vi "IECMemory.ProcCases.vi"(0 "i ref in":refnum<vi>, 1 "selector":string, 2 "Data":T2, 3 "call cluster":T6={"Object"="", "Selector"="", "CallType"=enum."synchronous", "Async Object"="", "Async Selector"="", "Data Descriptor"="", "Data"=[], "Error #"=0, "Expire"=0}, 5 "error in (no error)":errorcluster) -> (14 "i ref out":refnum<vi>, 17 "answer cluster":T6={"Object"="", "Selector"="", "CallType"=enum."synchronous", "Async Object"="", "Async Selector"="", "Data Descriptor"="", "Data"=[], "Error #"=0, "Expire"=0}, 19 "error out":errorcluster)   [LabVIEW 2014, in "IECMemory.lvlib"]
doc: "This method is called by a process from within the default case in the event loop. The methods of a class that are linked to events will be called from THIS method. Add your code here."
uses:
  IECMemory.lvlib
  CS_Core/BaseProcess/BaseProcess.lvlib
  CS_Core/CSSystem/CoreLib/CoreLib.lvlib
  CS_Core/CSSystem/CoreLib/CoreLib.string 2 byte array.vi
  CS_Core/CSSystem/CoreLib/CoreLib.byte array 2 string.vi
  CS_Core/CSSystem/CoreLib/CoreLib.byte array 2 int.vi
  CS_Core/CSSystem/CoreDefs/CoreDefs.call_type.ctl
  instr.lib/GPIB_Memory/Memory_Status.ctl
  CS_Lebit/LEBITDefs/LEBITDefs.MemDevInfo.ctl
  CS_Lebit/LEBITDefs/LEBITDefs.lvlib
  CS_Core/BaseProcess/BaseProcess.descriptor string definition.ctl
  CS_Core/CSSystem/CoreDefs/CoreDefs.rawDataType.ctl
  CS_Lebit/LEBITDefs/LEBITDefs.Memory.ctl
  CS_Lebit/LEBITDefs/LEBITDefs.Timetable.ctl
panel:
  in  "MemoryStatusBits":T1=[TRUE]
  in  "ms timeout (100)":i32=100
  in  "MemDevInfo":T3
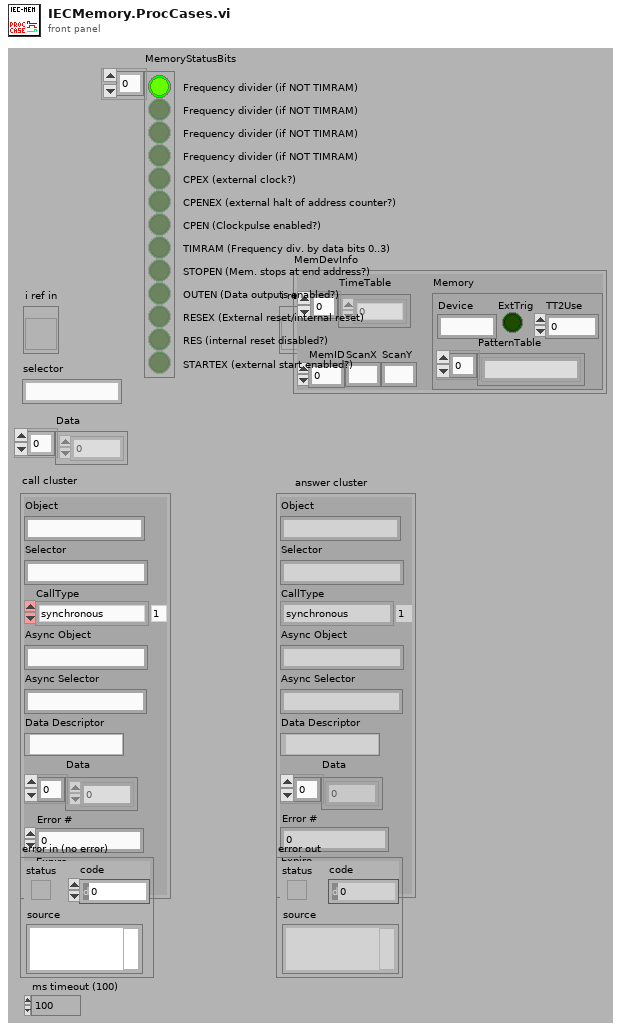
[diagram p1: front panel]
types:
  T1 = typedef "IECMemoryDriver.lvlib/Memory_Status.ctl" = bool[]
  T2 = typedef "CoreDefs.rawDataType.ctl" = i8[]
  T3 = typedef "LEBITDefs.lvlib/LEBITDefs.MemDevInfo.ctl" = cluster{"TimeTable":T4, "Memory":T5, "MemID":i32, "ScanX":string, "ScanY":string}
  T4 = typedef "LEBITDefs.lvlib/LEBITDefs.Timetable.ctl" = dbl[]
  T5 = typedef "LEBITDefs.lvlib/LEBITDefs.Memory.ctl" = cluster{"Device":string, "ExtTrig":bool, "TT2Use":i32, "PatternTable":string[]}
  T6 = typedef "CoreDefs.call_type.ctl" = cluster{"Object":string, "Selector":string, "CallType":enum16{"simple", "synchronous", "asynchronous"}, "Async Object":string, "Async Selector":string, "Data Descriptor":T7, "Data":T2, "Error #":i32, "Expire":u32}
  T7 = typedef "BaseProcess.lvlib/BaseProcess.descriptor string definition.ctl" = string
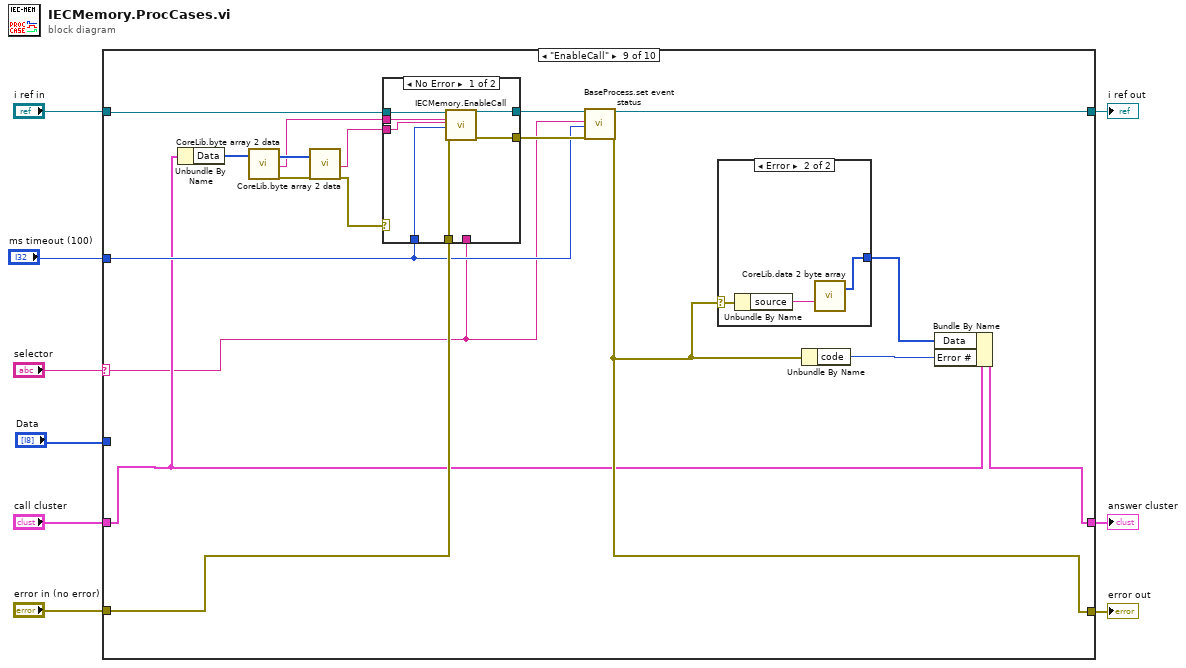
[diagram p0: block diagram]
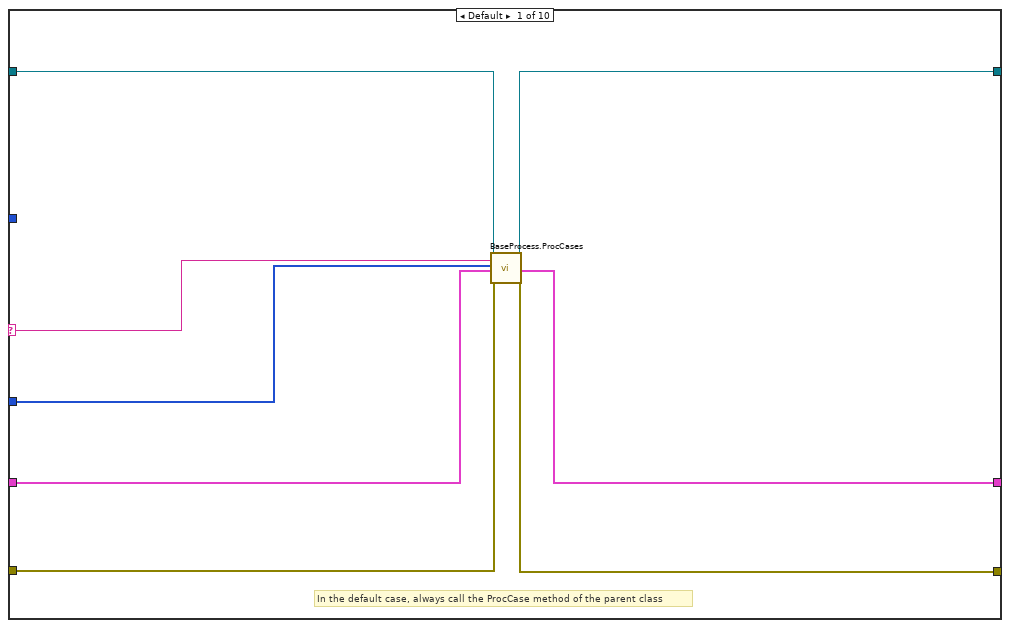
[diagram p2: hidden frame]
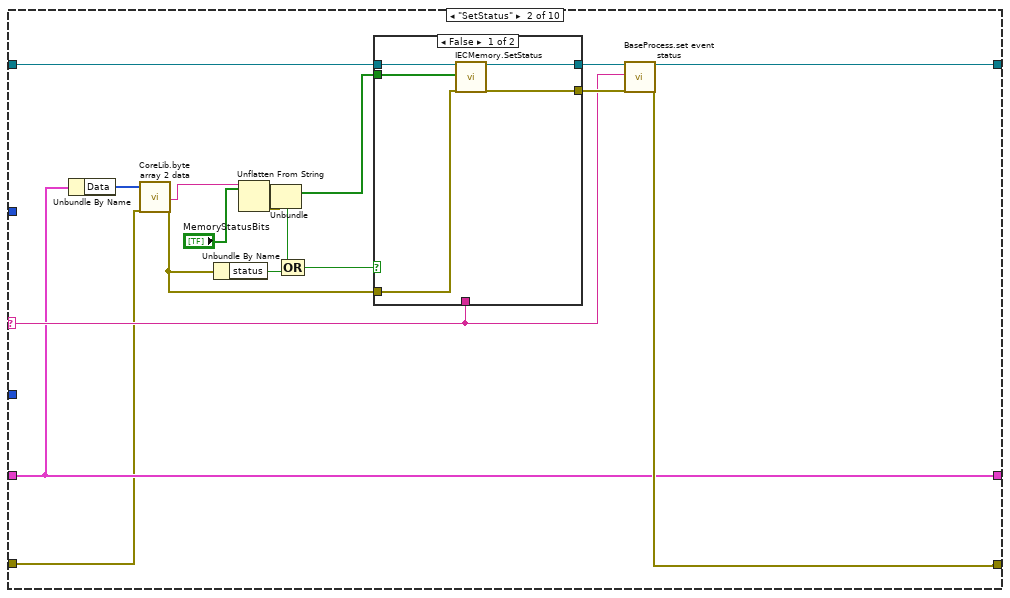
[diagram p3: hidden frame]
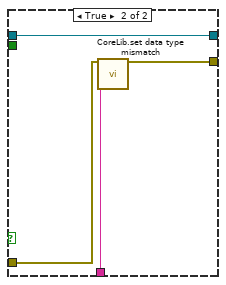
[diagram p4: hidden frame]
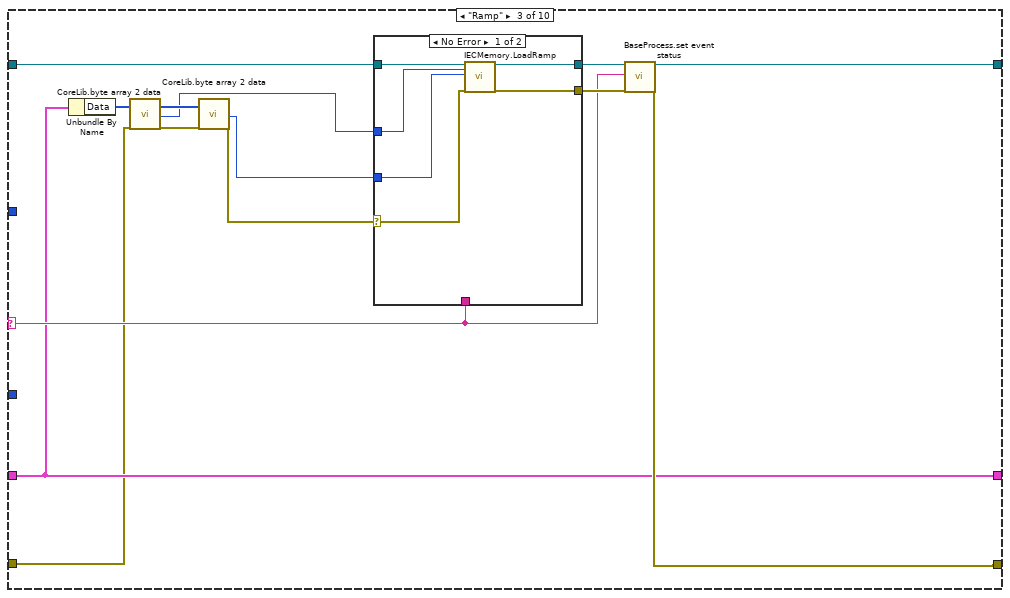
[diagram p5: hidden frame]
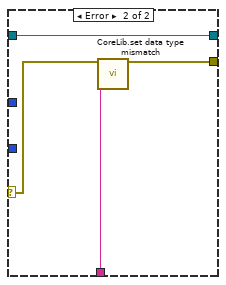
[diagram p6: hidden frame]
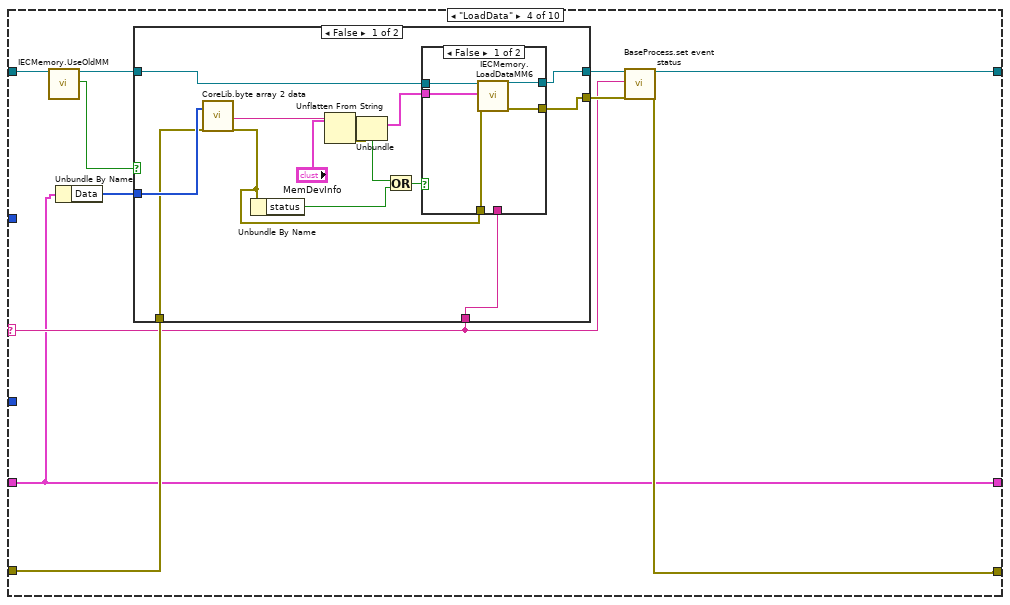
[diagram p7: hidden frame]
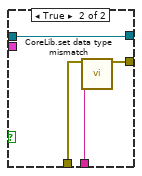
[diagram p8: hidden frame]
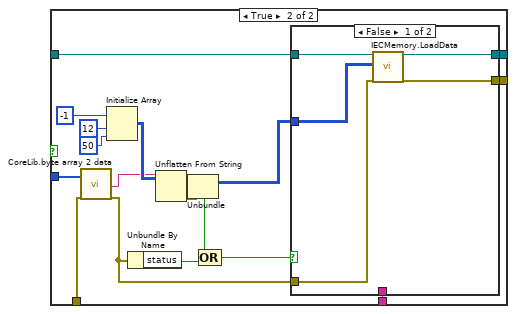
[diagram p9: hidden frame]
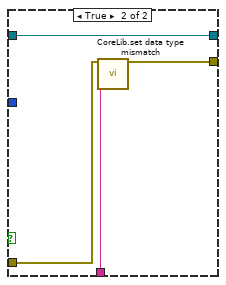
[diagram p10: hidden frame]
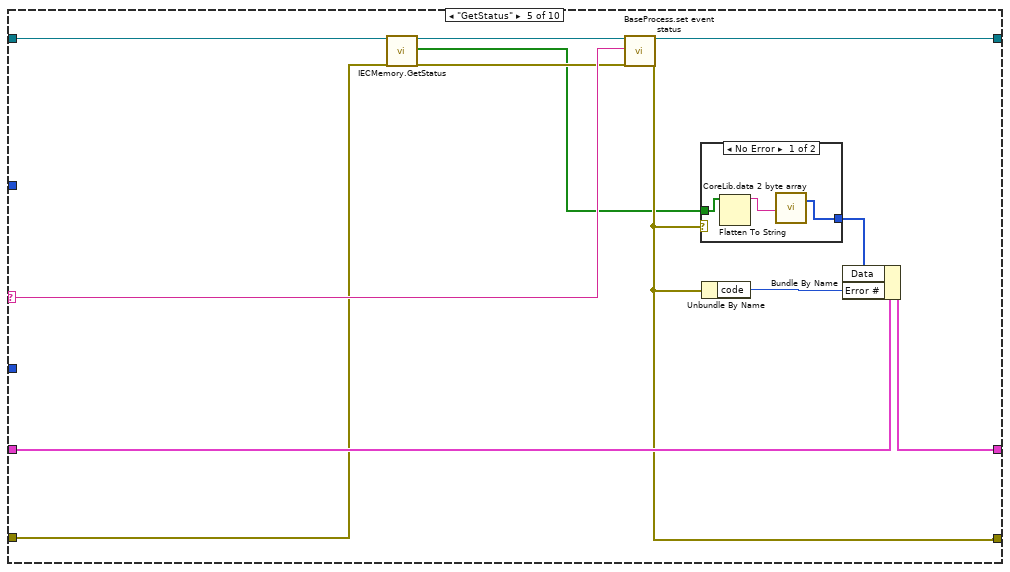
[diagram p11: hidden frame]
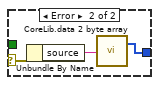
[diagram p12: hidden frame]
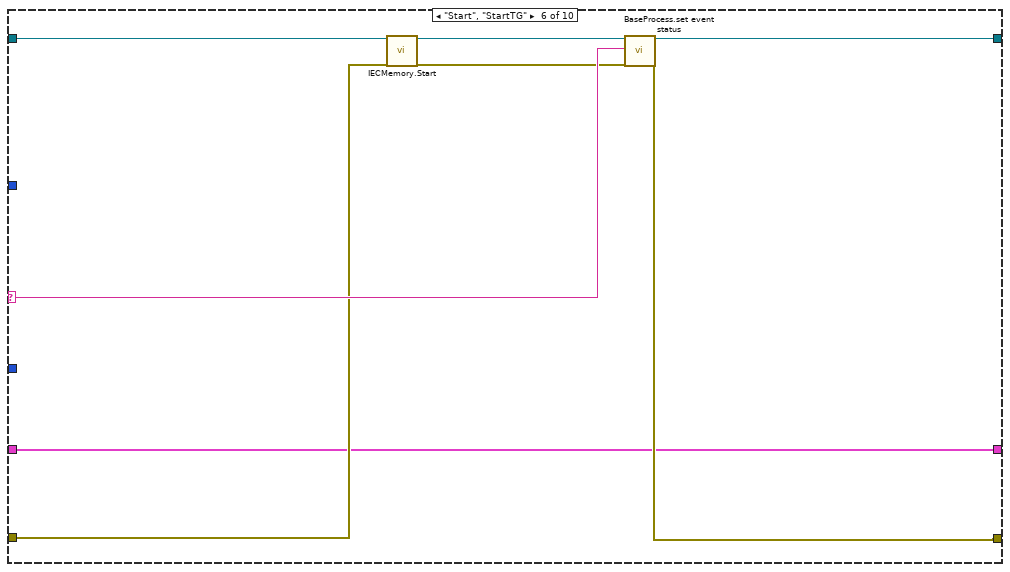
[diagram p13: hidden frame]
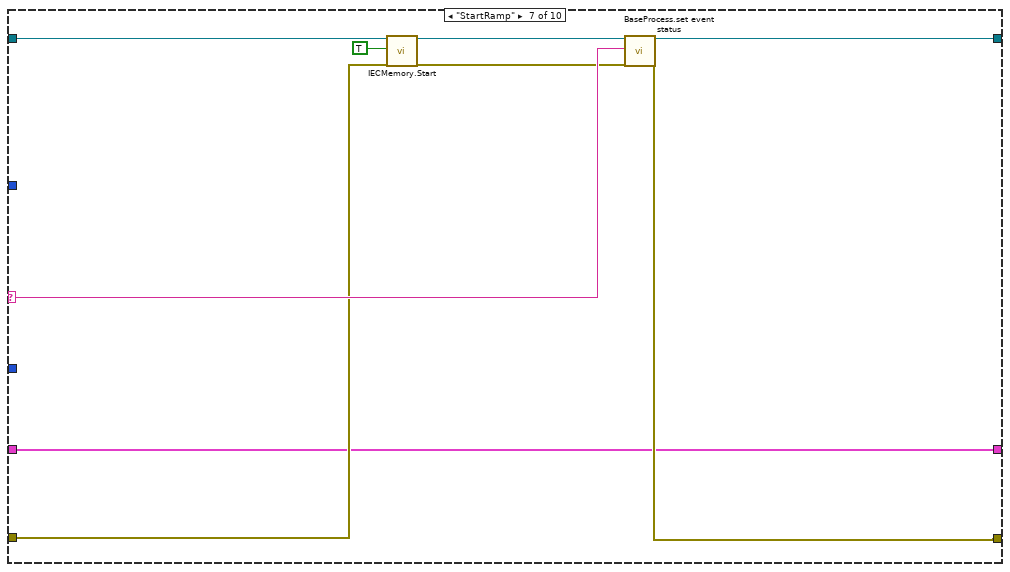
[diagram p14: hidden frame]
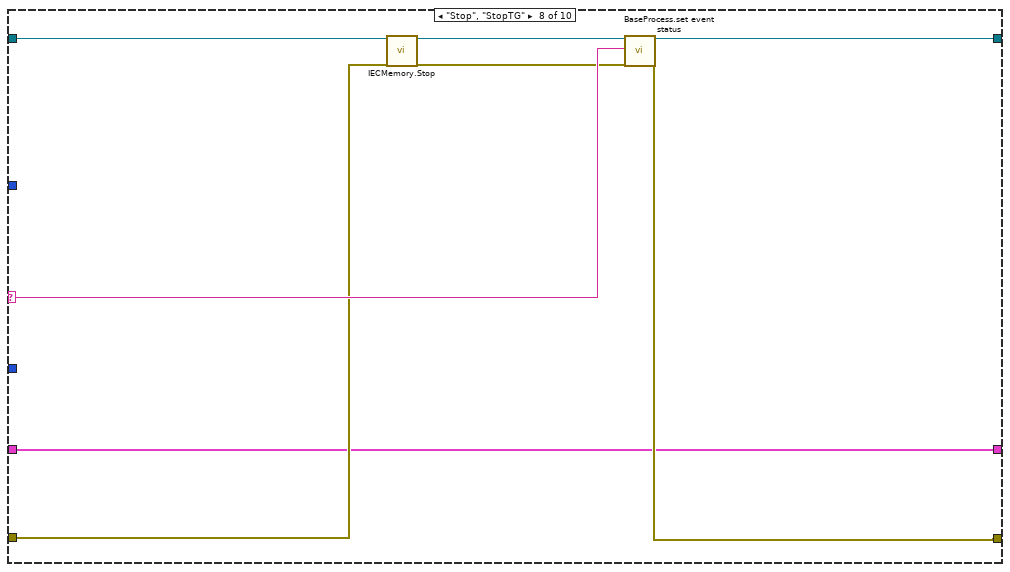
[diagram p15: hidden frame]
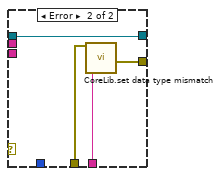
[diagram p16: hidden frame]
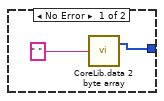
[diagram p17: hidden frame]
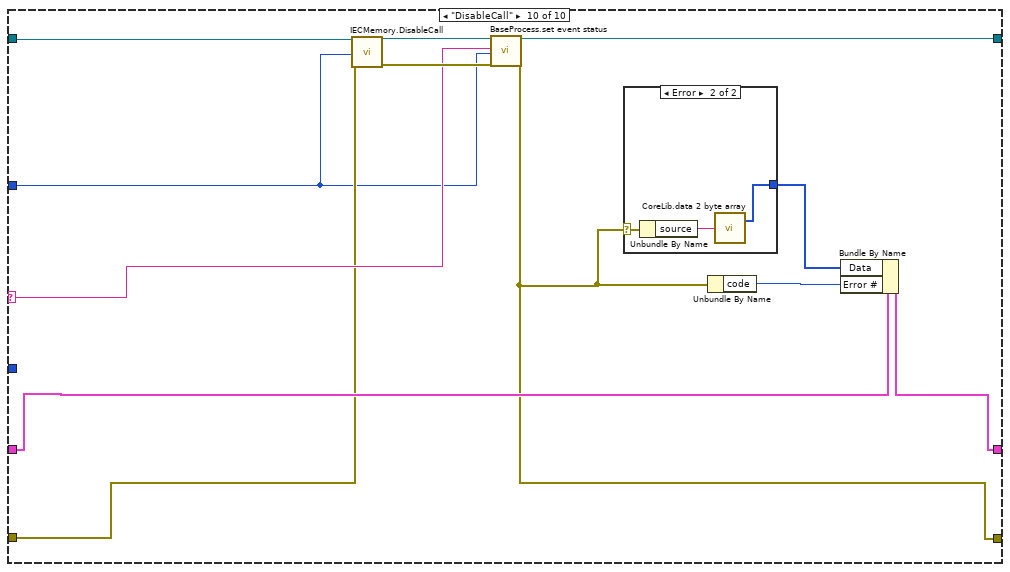
[diagram p18: hidden frame]
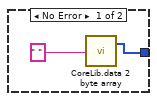
[diagram p19: hidden frame]
diagram:
  n1 = case shown="\"EnableCall\"" "selector" {
    selector: "selector" -> [w11 w29 w54 w75 w135 w152 w161 w169 w177 w210]
    tunnel: "Data" -> [w12 _ _ _ _ _ _ _ _ _]
    tunnel: "i ref in" -> [w10 w32 w57 w70 w133 w150 w159 w167 w184 w212]
    tunnel: [w17 w27 w53 w74 w134 w151 w160 w168 w182 w208] -> w5
    tunnel: "call cluster" -> [w13 w25 w51 w72 w138 w146 w155 w163 w178 w211]
    tunnel: [w14 w25 w51 w72 w137 w146 w155 w163 w181 w207] -> w8
    tunnel: "error in (no error)" -> [w16 w20 w44 w78 w132 w149 w158 w166 w183 w209]
    tunnel: [w15 w26 w52 w73 w136 w153 w162 w170 w180 w206] -> w3
    tunnel: "ms timeout (100)" -> [_ _ _ _ _ _ _ _ w179 w205]
    frame Default {
      # "In the default case, always call the ProcCase method of the parent class"
      n2 = call "BaseProcess.ProcCases.vi"("i ref in"=w10, "selector"=w11, "Data"=w12, "call cluster"=w13, "error in (no error)"=w16) -> ("i ref out"=w17:refnum<vi>, "answer cluster"=w14:T6, "error out"=w15:errorcluster)  [unwired: 12 in]
    }
    frame "SetStatus" {
      n3 = Unbundle By Name(w25) -> ("Data"=w24:T2)
      n4 = call-poly "CoreLib.byte array 2 data.vi"("byteArray"=w24, "error in (no error)"=w20) -> ("string"=w23:string, "error out"=w21:errorcluster)  [unwired: 15 in, 1 out]
      n5 = Unbundle By Name(w21) -> ("status"=w22:bool)
      n6 = Unflatten From String(type="MemoryStatusBits", binary string=w23) -> (value=w28:T1, error out=w18:errorcluster)  [unwired: 3 in, 1 out]
      n7 = Unbundle(w18) -> ("status"=w34:bool)  [unwired: 2 out]
      n8 = Compound Arithmetic op=OR(w34, w22) -> (w33:bool)
      n9 = case shown="False" w33 {
        tunnel: [w37 w43] -> w31
        tunnel: w32 -> [w38 w43]
        tunnel: [w36 w42] -> w30
        tunnel: w29 -> [_ w41]
        tunnel: w28 -> [w39 _]
        tunnel: w21 -> [w35 w40]
        frame False {
          n10 = call "IECMemory.SetStatus.vi"("i ref in"=w38, "MemoryStatusBits"=w39, "error in (no error)"=w35) -> ("i ref out"=w37:refnum<vi>, "error out"=w36:errorcluster)  [unwired: 14 in, 1 out]
        }
        frame True {
          n11 = call "CoreLib.set data type mismatch.vi"("error in (no error)"=w40, "error source"=w41) -> ("error out"=w42:errorcluster)  [unwired: 17 in]
        }
      }
      n12 = call "BaseProcess.set event status.vi"("i ref in"=w31, "EventStatus"=w29, "error in (no error)"=w30) -> ("i ref out"=w27:refnum<vi>, "error out"=w26:errorcluster)  [unwired: 14 in, 1 out]
    }
    frame "Ramp" {
      n13 = Unbundle By Name(w51) -> ("Data"=w50:T2)
      n14 = call-poly "CoreLib.byte array 2 data.vi"("byteArray"=w50, "error in (no error)"=w44) -> ("byteArray out"=w49:T2, "i32"=w45:i32, "error out"=w48:errorcluster)  [unwired: 15 in]
      n15 = call-poly "CoreLib.byte array 2 data.vi"("byteArray"=w49, "error in (no error)"=w48) -> ("i32"=w46:i32, "error out"=w47:errorcluster)  [unwired: 15 in, 1 out]
      n16 = case shown="No Error" w47 {
        selector: w47 -> [w58 w64]
        tunnel: [w62 w67] -> w56
        tunnel: w57 -> [w63 w67]
        tunnel: [w61 w66] -> w55
        tunnel: w54 -> [_ w65]
        tunnel: w45 -> [w59 _]
        tunnel: w46 -> [w60 _]
        frame No Error {
          n17 = call "IECMemory.LoadRamp.vi"("i ref in"=w63, "FirstStep"=w59, "SecondStep"=w60, "error in (no error)"=w58) -> ("i ref out"=w62:refnum<vi>, "error out"=w61:errorcluster)  [unwired: 13 in, 1 out]
        }
        frame Error {
          n18 = call "CoreLib.set data type mismatch.vi"("error in (no error)"=w64, "error source"=w65) -> ("error out"=w66:errorcluster)  [unwired: 17 in]
        }
      }
      n19 = call "BaseProcess.set event status.vi"("i ref in"=w56, "EventStatus"=w54, "error in (no error)"=w55) -> ("i ref out"=w53:refnum<vi>, "error out"=w52:errorcluster)  [unwired: 14 in, 1 out]
    }
    frame "LoadData" {
      n20 = call "IECMemory.UseOldMM.vi"("i ref in"=w70) -> ("i ref out"=w69:refnum<vi>, "Use Old MM?"=w68:bool)  [unwired: 15 in, 2 out]
      n21 = Unbundle By Name(w72) -> ("Data"=w71:T2)
      n22 = case shown="False" w68 {
        tunnel: w69 -> [w88 w116]
        tunnel: w78 -> [w81 w107]
        tunnel: [w90 w115] -> w77
        tunnel: [w89 w114] -> w76
        tunnel: w75 -> [w87 w113]
        tunnel: w71 -> [w86 w105]
        frame False {
          n23 = call-poly "CoreLib.byte array 2 data.vi"("byteArray"=w86, "error in (no error)"=w81) -> ("string"=w85:string, "error out"=w80:errorcluster)  [unwired: 15 in, 1 out]
          n24 = Unbundle By Name(w80) -> ("status"=w82:bool)
          n25 = Unflatten From String(type="MemDevInfo", binary string=w85) -> (value=w92:T3, error out=w79:errorcluster)  [unwired: 3 in, 1 out]
          n26 = Unbundle(w79) -> ("status"=w83:bool)  [unwired: 2 out]
          n27 = Or(x=w83, y=w82) -> (x .or. y?=w84:bool)
          n28 = case shown="False" w84 {
            tunnel: w88 -> [w97 w99]
            tunnel: w80 -> [w96 w100]
            tunnel: [w95 w99] -> w90
            tunnel: [w94 w101] -> w89
            tunnel: w92 -> [w93 _]
            tunnel: w87 -> [_ w98]
            frame False {
              n29 = call "IECMemory.LoadDataMM6.vi"("i ref in"=w97, "MemDevInfo"=w93, "error in (no error)"=w96) -> ("i ref out"=w95:refnum<vi>, "error out"=w94:errorcluster)  [unwired: 14 in, 1 out]
            }
            frame True {
              n30 = call "CoreLib.set data type mismatch.vi"("error in (no error)"=w100, "error source"=w98) -> ("error out"=w101:errorcluster)  [unwired: 17 in]
            }
          }
        }
        frame True {
          n31 = call-poly "CoreLib.byte array 2 data.vi"("byteArray"=w105, "error in (no error)"=w107) -> ("string"=w106:string, "error out"=w104:errorcluster)  [unwired: 15 in, 1 out]
          n32 = Initialize Array(-1 ("element"), 12 ("dimension size"), 50 ("dimension size")) -> (w108:i32[][])
          n33 = Unbundle By Name(w104) -> ("status"=w103:bool)
          n34 = Unflatten From String(type=w108, binary string=w106) -> (value=w112:i32[][], error out=w102:errorcluster)  [unwired: 3 in, 1 out]
          n35 = Unbundle(w102) -> ("status"=w118:bool)  [unwired: 2 out]
          n36 = Compound Arithmetic op=OR(w118, w103) -> (w117:bool)
          n37 = case shown="False" w117 {
            tunnel: [w122 w127] -> w115
            tunnel: w116 -> [w123 w127]
            tunnel: [w121 w126] -> w114
            tunnel: w113 -> [_ w125]
            tunnel: w112 -> [w120 _]
            tunnel: w104 -> [w119 w124]
            frame False {
              n38 = call "IECMemory.LoadData.vi"("i ref in"=w123, "MemoryTimingArray"=w120, "error in (no error)"=w119) -> ("i ref out"=w122:refnum<vi>, "error out"=w121:errorcluster)  [unwired: 14 in, 1 out]
            }
            frame True {
              n39 = call "CoreLib.set data type mismatch.vi"("error in (no error)"=w124, "error source"=w125) -> ("error out"=w126:errorcluster)  [unwired: 17 in]
            }
          }
        }
      }
      n40 = call "BaseProcess.set event status.vi"("i ref in"=w77, "EventStatus"=w75, "error in (no error)"=w76) -> ("i ref out"=w74:refnum<vi>, "error out"=w73:errorcluster)  [unwired: 14 in, 1 out]
    }
    frame "GetStatus" {
      n41 = call "IECMemory.GetStatus.vi"("i ref in"=w133, "error in (no error)"=w132) -> ("i ref out"=w131:refnum<vi>, "MemoryStatus"=w128:T1, "error out"=w130:errorcluster)  [unwired: 14 in, 1 out]
      n42 = call "BaseProcess.set event status.vi"("i ref in"=w131, "EventStatus"=w135, "error in (no error)"=w130) -> ("i ref out"=w134:refnum<vi>, "error out"=w136:errorcluster)  [unwired: 14 in, 1 out]
      n43 = case shown="No Error" w136 {
        selector: w136 -> [_ w145]
        tunnel: [w140 w143] -> w129
        tunnel: w128 -> [w142 _]
        frame No Error {
          n44 = Flatten To String(anything=w142) -> (data string=w141:string)  [unwired: 3 in, 2 out]
          n45 = call-poly "CoreLib.data 2 byte array.vi"("string"=w141) -> ("byteArray out"=w140:T2)  [unwired: 18 in]
        }
        frame Error {
          n46 = Unbundle By Name(w145) -> ("source"=w144:string)
          n47 = call-poly "CoreLib.data 2 byte array.vi"("string"=w144) -> ("byteArray out"=w143:T2)  [unwired: 18 in]
        }
      }
      n48 = Unbundle By Name(w136) -> ("code"=w139:i32)
      n49 = Bundle By Name(cluster=w138, "Data"=w129, "Error #"=w139) -> (w137:T6)
    }
    frame "Start", "StartTG" {
      n50 = call "IECMemory.Start.vi"("i ref in"=w150, "error in (no error)"=w149) -> ("i ref out"=w148:refnum<vi>, "error out"=w147:errorcluster)  [unwired: 15 in, 1 out]
      n51 = call "BaseProcess.set event status.vi"("i ref in"=w148, "EventStatus"=w152, "error in (no error)"=w147) -> ("i ref out"=w151:refnum<vi>, "error out"=w153:errorcluster)  [unwired: 14 in, 1 out]
    }
    frame "StartRamp" {
      n52 = call "IECMemory.Start.vi"("i ref in"=w159, "Ramp (F)"=TRUE, "error in (no error)"=w158) -> ("i ref out"=w157:refnum<vi>, "error out"=w156:errorcluster)  [unwired: 14 in, 1 out]
      n53 = call "BaseProcess.set event status.vi"("i ref in"=w157, "EventStatus"=w161, "error in (no error)"=w156) -> ("i ref out"=w160:refnum<vi>, "error out"=w162:errorcluster)  [unwired: 14 in, 1 out]
    }
    frame "Stop", "StopTG" {
      n54 = call "IECMemory.Stop.vi"("i ref in"=w167, "error in (no error)"=w166) -> ("i ref out"=w165:refnum<vi>, "error out"=w164:errorcluster)  [unwired: 15 in, 1 out]
      n55 = call "BaseProcess.set event status.vi"("i ref in"=w165, "EventStatus"=w169, "error in (no error)"=w164) -> ("i ref out"=w168:refnum<vi>, "error out"=w170:errorcluster)  [unwired: 14 in, 1 out]
    }
    frame "EnableCall" {
      n56 = Unbundle By Name(w178) -> ("Data"=w176:T2)
      n57 = call-poly "CoreLib.byte array 2 data.vi"("byteArray"=w176) -> ("byteArray out"=w174:T2, "string"=w172:string, "error out"=w175:errorcluster)  [unwired: 16 in]
      n58 = call-poly "CoreLib.byte array 2 data.vi"("byteArray"=w174, "error in (no error)"=w175) -> ("string"=w171:string, "error out"=w173:errorcluster)  [unwired: 15 in, 1 out]
      n59 = case shown="No Error" w173 {
        tunnel: [w195 w196] -> w186
        tunnel: [w194 w199] -> w185
        tunnel: w184 -> [w193 w196]
        tunnel: w183 -> [w192 w198]
        tunnel: w179 -> [w191 _]
        tunnel: w177 -> [_ w197]
        tunnel: w172 -> [w190 _]
        tunnel: w171 -> [w189 _]
        frame No Error {
          n60 = call "IECMemory.EnableCall.vi"("i ref in"=w193, "call process"=w190, "call event"=w189, "ms timeout (100)"=w191, "error in (no error)"=w192) -> ("i ref out"=w195:refnum<vi>, "error out"=w194:errorcluster)  [unwired: 12 in, 1 out]
        }
        frame Error {
          n61 = call "CoreLib.set data type mismatch.vi"("error in (no error)"=w198, "error source"=w197) -> ("error out"=w199:errorcluster)  [unwired: 17 in]
        }
      }
      n62 = call "BaseProcess.set event status.vi"("i ref in"=w186, "EventStatus"=w177, "ms timeout (10000)"=w179, "error in (no error)"=w185) -> ("i ref out"=w182:refnum<vi>, "error out"=w180:errorcluster)  [unwired: 13 in, 1 out]
      n63 = case shown="Error" w180 {
        selector: w180 -> [_ w204]
        tunnel: [w200 w202] -> w187
        frame No Error {
          n64 = call-poly "CoreLib.data 2 byte array.vi"("string"=" " ("source")) -> ("byteArray out"=w200:T2)  [unwired: 18 in]
        }
        frame Error {
          n65 = Unbundle By Name(w204) -> ("source"=w203:string)
          n66 = call-poly "CoreLib.data 2 byte array.vi"("string"=w203) -> ("byteArray out"=w202:T2)  [unwired: 18 in]
        }
      }
      n67 = Unbundle By Name(w180) -> ("code"=w188:i32)
      n68 = Bundle By Name(cluster=w178, "Data"=w187, "Error #"=w188) -> (w181:T6)
    }
    frame "DisableCall" {
      n69 = call "IECMemory.DisableCall.vi"("i ref in"=w212, "ms timeout (100)"=w205, "error in (no error)"=w209) -> ("i ref out"=w214:refnum<vi>, "error out"=w213:errorcluster)  [unwired: 14 in, 1 out]
      n70 = call "BaseProcess.set event status.vi"("i ref in"=w214, "EventStatus"=w210, "ms timeout (10000)"=w205, "error in (no error)"=w213) -> ("i ref out"=w208:refnum<vi>, "error out"=w206:errorcluster)  [unwired: 13 in, 1 out]
      n71 = case shown="Error" w206 {
        selector: w206 -> [_ w221]
        tunnel: [w217 w219] -> w215
        frame No Error {
          n72 = call-poly "CoreLib.data 2 byte array.vi"("string"=" " ("source")) -> ("byteArray out"=w217:T2)  [unwired: 18 in]
        }
        frame Error {
          n73 = Unbundle By Name(w221) -> ("source"=w220:string)
          n74 = call-poly "CoreLib.data 2 byte array.vi"("string"=w220) -> ("byteArray out"=w219:T2)  [unwired: 18 in]
        }
      }
      n75 = Unbundle By Name(w206) -> ("code"=w216:i32)
      n76 = Bundle By Name(cluster=w211, "Data"=w215, "Error #"=w216) -> (w207:T6)
    }
  }
  "answer cluster" <- w8
  "i ref out" <- w5
  "error out" <- w3
